vi "Error_Log.vi"(8 "error in (no error)":errorcluster) -> (0 "error out":errorcluster)   [LabVIEW 2019]
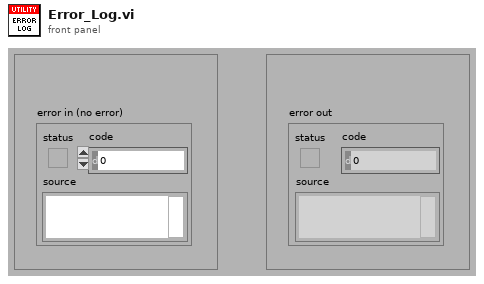
[diagram p1: front panel]
types:
  T1 = enum16{"open", "replace", "create", "open or create", "replace or create", "replace or create with confirmation"}
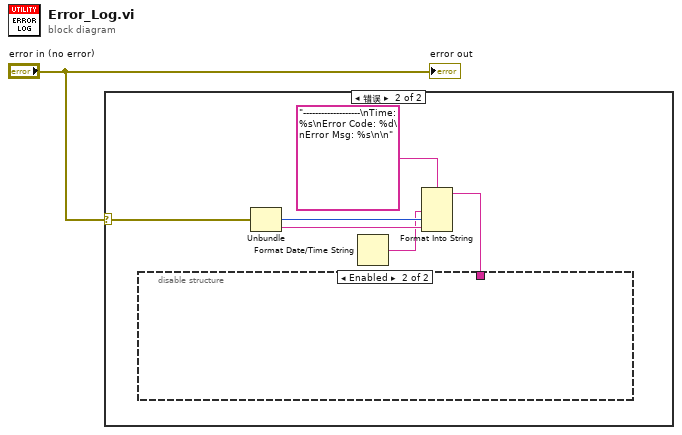
[diagram p0: block diagram]
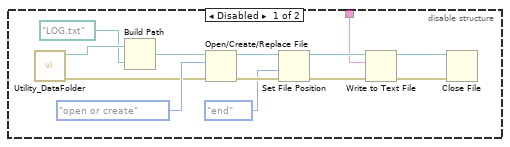
[diagram p3: hidden frame]
diagram:
  n1 = case shown="错误" "error in (no error)" {
    selector: "error in (no error)" -> [_ w7]
    frame No Error {
    }
    frame Error {
      n2 = Unbundle(w7) -> ("code"=w6:i32, "source"=w5:string)  [unwired: 1 out]
      n3 = Format Date/Time String() -> (date/time string=w2:string)  [unwired: 3 in]
      n4 = Format Into String(format string="-------------------\nTime: %s\nError Code: %d\nError Msg: %s\n\n", w2, w6, w5) -> (resulting string=w4:string)  [unwired: 2 in, 1 out]
      n5 = disable-structure shown="Enabled" {
        disable-tunnel: w4 -> [w12 _]
        frame Disabled {
          n6 = call "Utility_DataFolder.vi"() -> ("error out"=w8:errorcluster, "data folder"=w11:path)  [unwired: 10 in]
          n7 = Build Path(base path=w11, name or relative path=path "LOG.txt" ("path in")) -> (appended path=w9:path)
          n8 = Open/Create/Replace File(file path (use dialog)=w9, error in=w8, operation (0:open)=T1."open or create") -> (refnum out=w17:refnum<file>, error out=w19:errorcluster)  [unwired: 3 in, 1 out]
          n9 = Set File Position(refnum=w17, from (0:start)=enum16{"start", "end", "current"}."end", error in=w19) -> (refnum out=w16:refnum<file>, error out=w14:errorcluster)  [unwired: 1 in]
          n10 = Write to Text File(file (use dialog)=w16, text=w12, error in=w14) -> (refnum out=w15:refnum<file>, error out=w13:errorcluster)  [unwired: 1 in, 1 out]
          n11 = Close File(refnum=w15, error in=w13) -> ()  [unwired: 2 out]
        }
        frame Enabled {
        }
      }
    }
  }
  "error out" <- "error in (no error)"
